vi "WHILE and FOR LOOP.vi"() -> ()   [LabVIEW 2024]
panel:
  in  "ON / OFF":bool
  out "TEST 1":bool
  in  "Numeric":i32
  in  "Thermometer Control":dbl(slide) scale=0.0..100.0
  in  "Threshold":dbl
  out "Thermometer Indicator":dbl(slide) scale=0.0..100.0
  out "Overtemp":bool
  # "WHILE LOOP"
  # "FOR LOOP"
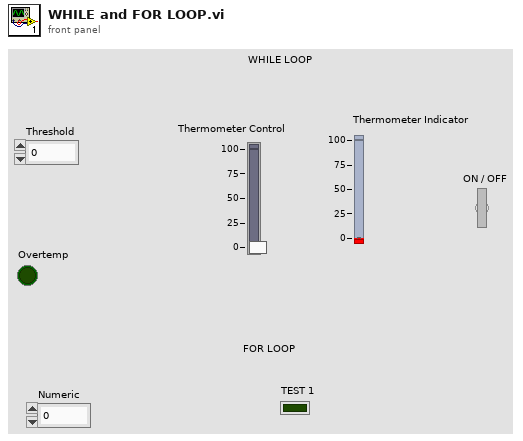
[diagram p1: front panel]
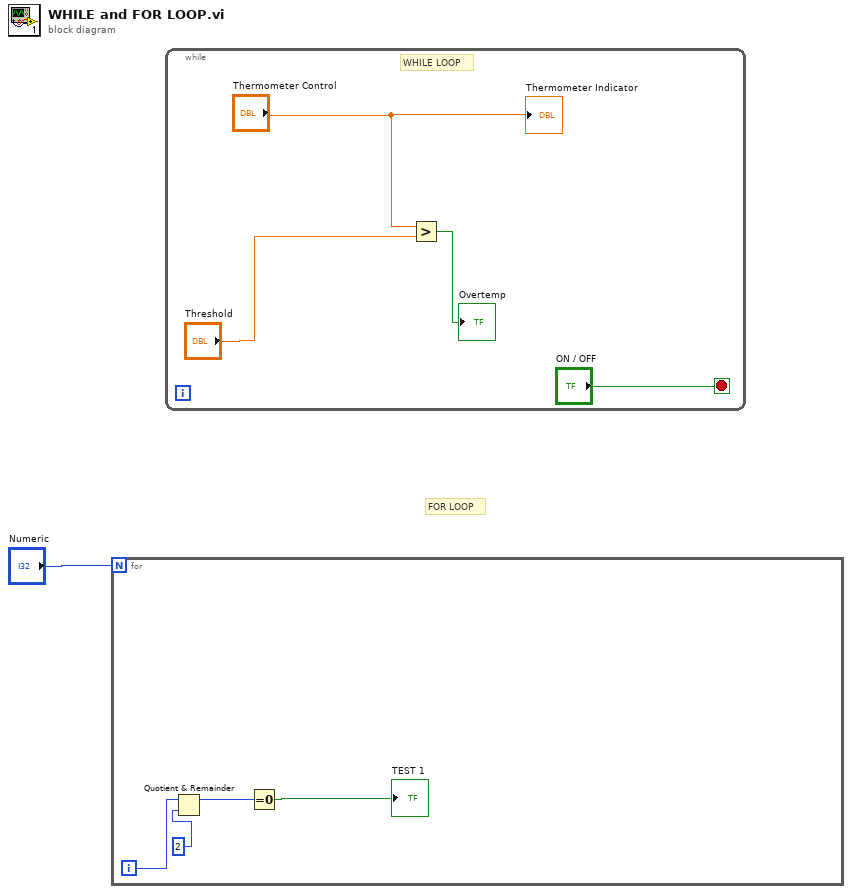
[diagram p0: block diagram]
diagram:
  # "FOR LOOP"
  n1 = for {
    N: "Numeric" -> [_]
    i -> [w5]
    n2 = Quotient & Remainder(x=w5, y=2) -> (x-y*floor(x/y)=w3:i32)  [unwired: 1 out]
    n3 = Equal To 0?(x=w3) -> (x = 0?=→"TEST 1":bool)
  }
  n4 = while {
    stop <- "ON / OFF" stop-if-true
    # "WHILE LOOP"
    n5 = Greater?(x="Thermometer Control", y="Threshold") -> (0:→"Overtemp":bool)
    "Thermometer Indicator" <- "Thermometer Control"
  }
